vi "integrate.vi"(10 "Numeric":dbl, 11 "Wrapper Out":u64) -> (1 "Length":i32, 2 "Spectrum Values":dbl[](array[numeric]), 3 "WL Values":dbl[](array[numeric]))   [LabVIEW 2020]
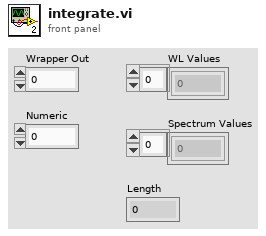
[diagram p1: front panel]
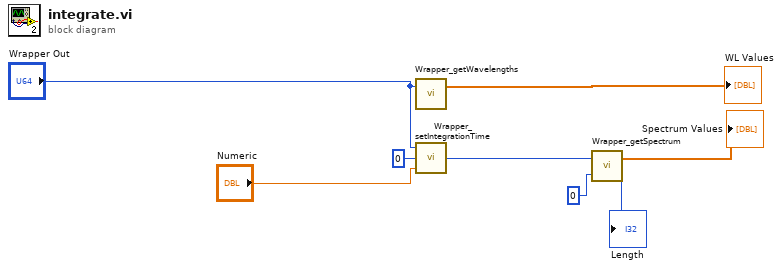
[diagram p0: block diagram]
diagram:
  n1 = call "Wrapper_getWavelengths.vi"("Wrapper"="Wrapper Out") -> ("WL Values"=→"WL Values":dbl[])  [unwired: 1 in, 1 out]
  n2 = call "Wrapper_setIntegrationTime.vi"("Integration Time"="Numeric", "Spectrometer Index"=0 ("Index"), "Wrapper In"="Wrapper Out") -> ("Wrapper Out"=w4:u32)
  n3 = call "Wrapper_getSpectrum.vi"("Index"=0, "Wrapper"=w4) -> ("Length"=→"Length":i32, "Spectrum Values"=→"Spectrum Values":dbl[])
